vi "NIReadMethod.vi"(8 "save?":bool=TRUE, 10 "Digitizer Settings":T1={"Digitizer delay (us) "=0.0, "rf points per line"=2048, "lines per plane"=128, "Samp Rate (Hz)"=100000000.0, "Additional dig delay (us)"=0.0, "Voltage Scale"=0.4, "Pre-Looks"=0, "Offset delay (us)"=0.0, "bits A/D"=8, "Avg Num"=1, "DigTimeOut"=5.0, "Rel Dig Delay"=0.0, "Dig Ch"=0, "LeCroyCluster"={"LeCroy Channels"=[TRUE, FALSE, FALSE, FALSE], "LC read pt offset"=0.0, "Sweep Avg"=FALSE}, "Main Digitizer"=enum."NI Digitizer", "Dig Config"=enum."Single channel", "Digitizer ID Cluster"={"Acqiris/Alazar/SP ID"=[], "NI Instr Handles"=[], "LeCroy VISA"="", "GaGe Handle"={"Handle"=0, "Sample size"=0, "Resolution"=0, "Offset"=0, "Channels"=0, "Boards"=0}, "ATS Ref"="ATS9350", "Acqiris Address"=["PCI::INSTR0"], "ADQRef"=refnum, "adq_cu_ptr"=refnum}, "Trigger Settings"={"Trig Source"=1, "Trig Coupling"=0, "Trig Slope"=0, "Level (mV)"=1500.0}, "Bulk Acq"=FALSE, "Bulk Start Indexes"=[], "Data Ref RF"=refnum, "NI ID/Channel"=[], "Total Dig CH"=1, "Xtra Ann Trig delay (us)"=10.0, "Fix Z Delay?"=FALSE, "One Way Transmission?"=FALSE, "Data Ref Log"=refnum} {"Trigger Settings"."Trig Slope" items=["Positive", "Negative"]; "Trigger Settings"."Level (mV)" format="%.2f"; "Trigger Settings"."Trig Coupling" items=["DC 1 MOhm", "AC 1 MOhm", "DC 50 Ohm", "AC 50 Ohm"]; "Trigger Settings"."Trig Source" items=["Chan 1", "External"]; "Rel Dig Delay" format="%.2f"; "DigTimeOut" format="%.2f"; "Avg Num" min=1; "Offset delay (us)" format="%.2f"; "Additional dig delay (us)" format="%.2f"; "Digitizer delay (us)" format="%.2f"}, 11 "Synth Foc?":bool) -> (3 "Read Method":T5=enum."5-Ch Pulser Synth Focus")   [LabVIEW 2022 SP3]
uses:
  NIReadList.ctl
  -DigitizerRoutines/DigitizerSettings.ctl
  -DigitizerRoutines/Digitizer.ctl
  -DigitizerRoutines/DigConfig.ctl
  -DigitizerRoutines/DigitizerID.ctl
  C:/Windows/System32/ADQAPI_dotNet_helper.dll
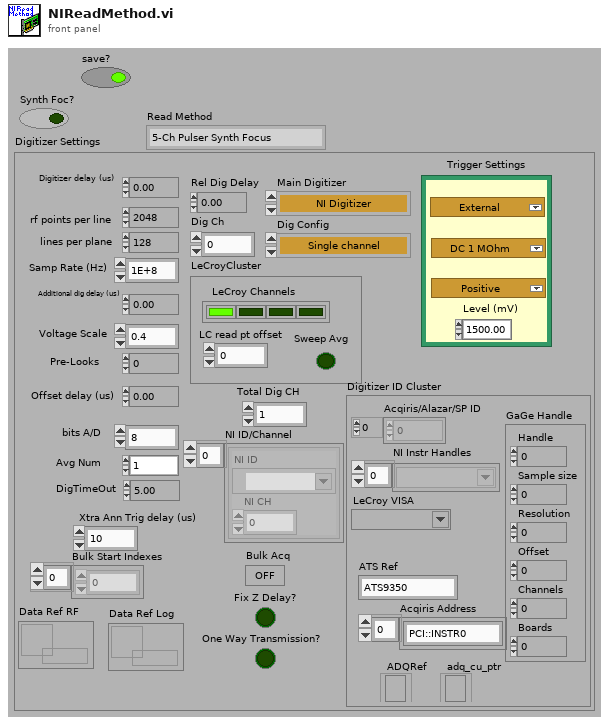
[diagram p1: front panel]
types:
  T1 = typedef "DigitizerSettings.ctl" = cluster{"Digitizer delay (us) ":dbl, "rf points per line":i32, "lines per plane":i32, "Samp Rate (Hz)":dbl, "Additional dig delay (us)":dbl, "Voltage Scale":dbl, "Pre-Looks":i32, "Offset delay (us)":dbl, "bits A/D":i8, "Avg Num":i32, "DigTimeOut":sgl, "Rel Dig Delay":sgl, "Dig Ch":i32, "LeCroyCluster":cluster{"LeCroy Channels":bool[], "LC read pt offset":dbl, "Sweep Avg":bool}, "Main Digitizer":T2, "Dig Config":T3, "Digitizer ID Cluster":T4, "Trigger Settings":cluster{"Trig Source":u16, "Trig Coupling":u16, "Trig Slope":u16, "Level (mV)":dbl}, "Bulk Acq":bool, "Bulk Start Indexes":i32[], "Data Ref RF":refnum<data-value>, "NI ID/Channel":cluster{"NI ID":refnum<k15>, "NI CH":i32}[], "Total Dig CH":i32, "Xtra Ann Trig delay (us)":dbl, "Fix Z Delay?":bool, "One Way Transmission?":bool, "Data Ref Log":refnum<data-value>}
  T2 = typedef "Digitizer.ctl" = enum16{"Acqiris Digitizer", "NI Digitizer", "LeCroy", "GaGe", "AlazarTech", "No Digitizer", "Teledyne"}
  T3 = typedef "DigConfig.ctl" = enum16{"Single channel", "2 Chans w/ 2 Acqiris", "2 Chans w/ 1 Acqiris", "5-CH Pulser New", "5-CH pulser w/ ann array", "5-pass style ann array", "Empty"}
  T4 = typedef "DigitizerID.ctl" = cluster{"Acqiris/Alazar/SP ID":u32[], "NI Instr Handles":refnum<k15>[], "LeCroy VISA":refnum<visa-resource-name>, "GaGe Handle":cluster{"Handle":u32, "Sample size":u32, "Resolution":i32, "Offset":i32, "Channels":u32, "Boards":u32}, "ATS Ref":string, "Acqiris Address":string[], "ADQRef":refnum<k24>, "adq_cu_ptr":refnum<k24>}
  T5 = typedef "NIReadList.ctl" = enum16{"Standard File Dump", "Bulk Acq File Dump", "Send data out", "Synth Focus Each Pass", "Synth Focus Bulk", "5-Ch Pulser File Dump", "5-Ch Pulser Synth Focus", "5-Ch Pulser File Dump AVG"}
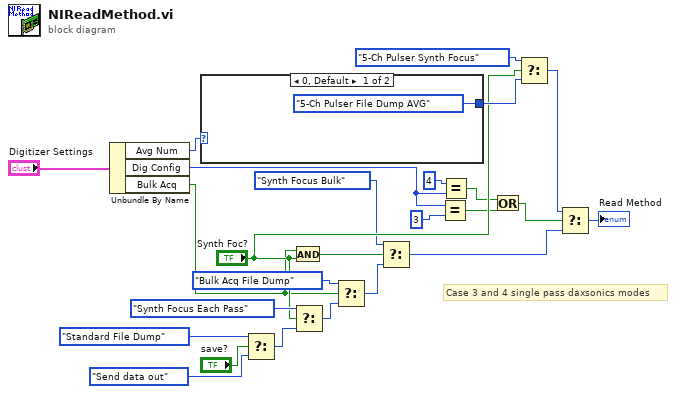
[diagram p0: block diagram]
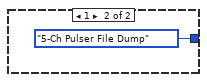
[diagram p2: hidden frame]
diagram:
  # "Case 3 and 4 single pass daxsonics modes"
  n1 = Unbundle By Name("Digitizer Settings") -> ("Avg Num"=w7:i32, "Dig Config"=w4:T3, "Bulk Acq"=w6:bool)
  n2 = case shown="0, Default" w7 {
    tunnel: [NIReadList."5-Ch Pulser File Dump AVG" ("Read Method") NIReadList."5-Ch Pulser File Dump" ("Read Method")] -> w14
    frame 0, Default {
    }
    frame 1 {
    }
  }
  n3 = Select(t=NIReadList."Standard File Dump" ("Read Method"), s="save?", f=NIReadList."Send data out" ("Read Method")) -> (s? t:f=w22:T5)
  n4 = And(x=w6, y="Synth Foc?") -> (x .and. y?=w12:bool)
  n5 = Select(t=NIReadList."Synth Focus Each Pass" ("Read Method"), s="Synth Foc?", f=w22) -> (s? t:f=w23:T5)
  n6 = Select(t=NIReadList."Bulk Acq File Dump" ("Read Method"), s=w6, f=w23) -> (s? t:f=w11:T5)
  n7 = Select(t=NIReadList."Synth Focus Bulk" ("Read Method"), s=w12, f=w11) -> (s? t:f=w10:T5)
  n8 = Equal?(x=w4, y=3) -> (x = y?=w3:bool)
  n9 = Equal?(x=4, y=w4) -> (x = y?=w2:bool)
  n10 = Or(x=w2, y=w3) -> (x .or. y?=w1:bool)
  n11 = Select(t=NIReadList."5-Ch Pulser Synth Focus" ("Read Method"), s="Synth Foc?", f=w14) -> (s? t:f=w24:T5)
  n12 = Select(t=w24, s=w1, f=w10) -> (s? t:f=→"Read Method":T5)
